vi "ReadAttribute_YCC.vi"() -> ()   [LabVIEW 2014]
uses:
  <vilib>/vision/driver/IMAQdx.llb/IMAQdx Attribute Type.ctl
  <vilib>/vision/driver/IMAQdx.llb/IMAQdx Attribute Visibility.ctl
  <vilib>/userDefined/High Color/IMAQdx.ctl
  <vilib>/vision/driver/IMAQdx.llb/IMAQdx Camera Control Mode.ctl
  <vilib>/vision/driver/NI_Vision_Acquisition_Software.lvlib
  <resource>/objmgr/imaqdx.rc
panel:
  out "Array 2":string[](array[string])=["AcquisitionAttributes::AdvancedGenicam::CommandTimeout", "AcquisitionAttributes::AdvancedGenicam::EventQueueDepth", "AcquisitionAttributes::AdvancedGenicam::EventsEnabled", "AcquisitionAttributes::AdvancedGenicam::EventsSupported", "AcquisitionAttributes::AdvancedGenicam::IgnoreCameraValidationErrors", "AcquisitionAttributes::AdvancedUSB3Vision::ActualMaximumPayloadTransferSize", "AcquisitionAttributes::AdvancedUSB3Vision::RequiredPayloadSizeAlignment", "AcquisitionAttributes::Bayer::Algorithm", "AcquisitionAttributes::Bayer::GainB", "AcquisitionAttributes::Bayer::GainG", "AcquisitionAttributes::Bayer::GainR", "AcquisitionAttributes::Bayer::Pattern", "AcquisitionAttributes::ChunkDataDecoding::ChunkDataDecodingEnabled", "AcquisitionAttributes::ChunkDataDecoding::MaximumChunkCopySize", "CameraAttributes::SequencerControl::SequencerMode", "CameraAttributes::SequencerControl::SequencerSetActive", "CameraAttributes::SequencerControl::SequencerConfigurationMode", "CameraAttributes::SequencerControl::SequencerSetStart", "CameraAttributes::SequencerControl::SequencerSetSelector", "CameraAttributes::SequencerControl::SequencerSetLoad", "CameraAttributes::SequencerControl::SequencerSetSave", "CameraAttributes::SequencerControl::SequencerPathSelector", "CameraAttributes::SequencerControl::SequencerSetNext", "CameraAttributes::SequencerControl::SequencerTriggerSource", "CameraAttributes::SequencerControl::SequencerTriggerActivation", "CameraAttributes::ImageFormatControl::SensorWidth", "CameraAttributes::ImageFormatControl::SensorHeight", "CameraAttributes::ImageFormatControl::WidthMax", "CameraAttributes::ImageFormatControl::HeightMax", "CameraAttributes::ImageFormatControl::Width", "CameraAttributes::ImageFormatControl::Height", "CameraAttributes::ImageFormatControl::OffsetX", "CameraAttributes::ImageFormatControl::OffsetY", "CameraAttributes::ImageFormatControl::CenterX", "CameraAttributes::ImageFormatControl::CenterY", "CameraAttributes::ImageFormatControl::BinningHorizontalMode", "CameraAttributes::ImageFormatControl::BinningHorizontal", "CameraAttributes::ImageFormatControl::BinningVerticalMode", "CameraAttributes::ImageFormatControl::BinningVertical", "CameraAttributes::ImageFormatControl::ReverseX", "CameraAttributes::ImageFormatControl::ReverseY", "CameraAttributes::ImageFormatControl::PixelFormat", "CameraAttributes::ImageFormatControl::PixelSize", "CameraAttributes::ImageFormatControl::PixelColorFilter", "CameraAttributes::ImageFormatControl::PixelDynamicRangeMin", "CameraAttributes::ImageFormatControl::PixelDynamicRangeMax", "CameraAttributes::ImageFormatControl::TestImageSelector", "CameraAttributes::ImageFormatControl::TestImageResetAndHold", "CameraAttributes::ImageFormatControl::ROIZoneSelector", "CameraAttributes::ImageFormatControl::ROIZoneMode", "CameraAttributes::ImageFormatControl::ROIZoneSize", "CameraAttributes::ImageFormatControl::ROIZoneOffset", "CameraAttributes::AnalogControl::GainAuto", "CameraAttributes::AnalogControl::GainSelector", "CameraAttributes::AnalogControl::Gain", "CameraAttributes::AnalogControl::BlackLevelSelector", "CameraAttributes::AnalogControl::BlackLevel", "CameraAttributes::AnalogControl::Gamma", "CameraAttributes::AnalogControl::DigitalShift", "CameraAttributes::ImageQualityControl::PGIControl::PgiMode", "CameraAttributes::ImageQualityControl::PGIControl::NoiseReduction", "CameraAttributes::ImageQualityControl::PGIControl::SharpnessEnhancement", "CameraAttributes::ImageQualityControl::ColorTransformationValue", "CameraAttributes::AcquisitionControl::AcquisitionMode", "CameraAttributes::AcquisitionControl::ShutterMode", "CameraAttributes::AcquisitionControl::ExposureAuto", "CameraAttributes::AcquisitionControl::ExposureMode", "CameraAttributes::AcquisitionControl::ExposureTime", "CameraAttributes::AcquisitionControl::ExposureOverlapTimeMode", "CameraAttributes::AcquisitionControl::ExposureOverlapTimeMax", "CameraAttributes::AcquisitionControl::AcquisitionBurstFrameCount", "CameraAttributes::AcquisitionControl::TriggerSelector", "CameraAttributes::AcquisitionControl::TriggerMode", "CameraAttributes::AcquisitionControl::TriggerSoftware", "CameraAttributes::AcquisitionControl::TriggerSource", "CameraAttributes::AcquisitionControl::TriggerActivation", "CameraAttributes::AcquisitionControl::TriggerDelay", "CameraAttributes::AcquisitionControl::AcquisitionFrameRateEnable", "CameraAttributes::AcquisitionControl::AcquisitionFrameRate", "CameraAttributes::AcquisitionControl::ResultingFrameRate", "CameraAttributes::AcquisitionControl::SensorReadoutTime", "CameraAttributes::AcquisitionControl::AcquisitionStatusSelector", "CameraAttributes::AcquisitionControl::AcquisitionStatus", "CameraAttributes::AutoFunctionControl::AutoTargetBrightness", "CameraAttributes::AutoFunctionControl::AutoFunctionProfile", "CameraAttributes::AutoFunctionControl::AutoGainLowerLimit", "CameraAttributes::AutoFunctionControl::AutoGainUpperLimit", "CameraAttributes::AutoFunctionControl::AutoExposureTimeLowerLimit", "CameraAttributes::AutoFunctionControl::AutoExposureTimeUpperLimit", "CameraAttributes::AutoFunctionControl::AutoFunctionROIControl::AutoFunctionROISelector", "CameraAttributes::AutoFunctionControl::AutoFunctionROIControl::AutoFunctionROIWidth", "CameraAttributes::AutoFunctionControl::AutoFunctionROIControl::AutoFunctionROIHeight", "CameraAttributes::AutoFunctionControl::AutoFunctionROIControl::AutoFunctionROIOffsetX", "CameraAttributes::AutoFunctionControl::AutoFunctionROIControl::AutoFunctionROIOffsetY", "CameraAttributes::AutoFunctionControl::AutoFunctionROIControl::AutoFunctionROIUseBrightness", "CameraAttributes::AutoFunctionControl::AutoFunctionROIControl::AutoFunctionROIUseWhiteBalance", "CameraAttributes::LUTControl::LUTSelector", "CameraAttributes::LUTControl::LUTEnable", "CameraAttributes::LUTControl::LUTIndex", "CameraAttributes::LUTControl::LUTValue", "CameraAttributes::DigitalIOControl::LineSelector", "CameraAttributes::DigitalIOControl::LineMode", "CameraAttributes::DigitalIOControl::LineFormat", "CameraAttributes::DigitalIOControl::LineLogic", "CameraAttributes::DigitalIOControl::LineSource", "CameraAttributes::DigitalIOControl::LineInverter", "CameraAttributes::DigitalIOControl::LineDebouncerTime", "CameraAttributes::DigitalIOControl::LineMinimumOutputPulseWidth", "CameraAttributes::DigitalIOControl::LineOverloadStatus", "CameraAttributes::DigitalIOControl::LineStatus", "CameraAttributes::DigitalIOControl::LineStatusAll", "CameraAttributes::DigitalIOControl::UserOutputSelector", "CameraAttributes::DigitalIOControl::UserOutputValue", "CameraAttributes::DigitalIOControl::UserOutputValueAll", "CameraAttributes::SoftwareSignalControl::SoftwareSignalSelector", "CameraAttributes::SoftwareSignalControl::SoftwareSignalPulse", "CameraAttributes::CounterAndTimerControl::TimerSelector", "CameraAttributes::CounterAndTimerControl::TimerDuration", "CameraAttributes::CounterAndTimerControl::TimerDelay", "CameraAttributes::CounterAndTimerControl::TimerTriggerSource", "CameraAttributes::CounterAndTimerControl::CounterSelector", "CameraAttributes::CounterAndTimerControl::CounterEventSource", "CameraAttributes::CounterAndTimerControl::CounterResetSource", "CameraAttributes::CounterAndTimerControl::CounterResetActivation", "CameraAttributes::CounterAndTimerControl::CounterReset", "CameraAttributes::CounterAndTimerControl::CounterDuration", "CameraAttributes::ChunkDataControl::ChunkModeActive", "CameraAttributes::ChunkDataControl::ChunkSelector", "CameraAttributes::ChunkDataControl::ChunkEnable", "CameraAttributes::ChunkDataControl::ChunkGainSelector", "CameraAttributes::ChunkDataControl::ChunkGain", "CameraAttributes::ChunkDataControl::ChunkExposureTime", "CameraAttributes::ChunkDataControl::ChunkTimestamp", "CameraAttributes::ChunkDataControl::ChunkLineStatusAll", "CameraAttributes::ChunkDataControl::ChunkCounterSelector", "CameraAttributes::ChunkDataControl::ChunkCounterValue", "CameraAttributes::ChunkDataControl::ChunkSequencerSetActive", "CameraAttributes::ChunkDataControl::ChunkPayloadCRC16", "CameraAttributes::ChunkDataControl::ChunkData::ChunkGainSelector", "CameraAttributes::ChunkDataControl::ChunkData::ChunkGain", "CameraAttributes::ChunkDataControl::ChunkData::ChunkExposureTime", "CameraAttributes::ChunkDataControl::ChunkData::ChunkTimestamp", "CameraAttributes::ChunkDataControl::ChunkData::ChunkLineStatusAll", "CameraAttributes::ChunkDataControl::ChunkData::ChunkCounterSelector", "CameraAttributes::ChunkDataControl::ChunkData::ChunkCounterValue", "CameraAttributes::ChunkDataControl::ChunkData::ChunkSequencerSetActive", "CameraAttributes::ChunkDataControl::ChunkData::ChunkPayloadCRC16", "CameraAttributes::EventControl::EventSelector", "CameraAttributes::EventControl::EventNotification", "CameraAttributes::EventControl::EventExposureEndData::EventExposureEnd", "CameraAttributes::EventControl::EventExposureEndData::EventExposureEndTimestamp", "CameraAttributes::EventControl::EventExposureEndData::EventExposureEndFrameID", "CameraAttributes::EventControl::EventFrameStartData::EventFrameStart", "CameraAttributes::EventControl::EventFrameStartData::EventFrameStartTimestamp", "CameraAttributes::EventControl::EventFrameStartData::EventFrameStartFrameID", "CameraAttributes::EventControl::EventFrameBurstStartData::EventFrameBurstStart", "CameraAttributes::EventControl::EventFrameBurstStartData::EventFrameBurstStartTimestamp", "CameraAttributes::EventControl::EventFrameBurstStartData::EventFrameBurstStartFrameID", "CameraAttributes::EventControl::EventFrameStartOvertriggerData::EventFrameStartOvertrigger", "CameraAttributes::EventControl::EventFrameStartOvertriggerData::EventFrameStartOvertriggerTimestamp", "CameraAttributes::EventControl::EventFrameStartOvertriggerData::EventFrameStartOvertriggerFrameID", "CameraAttributes::EventControl::EventFrameBurstStartOvertriggerData::EventFrameBurstStartOvertrigger", "CameraAttributes::EventControl::EventFrameBurstStartOvertriggerData::EventFrameBurstStartOvertriggerTimestamp", "CameraAttributes::EventControl::EventFrameBurstStartOvertriggerData::EventFrameBurstStartOvertriggerFrameID", "CameraAttributes::EventControl::EventCriticalTemperatureData::EventCriticalTemperature", "CameraAttributes::EventControl::EventCriticalTemperatureData::EventCriticalTemperatureTimestamp", "CameraAttributes::EventControl::EventOverTemperatureData::EventOverTemperature", "CameraAttributes::EventControl::EventOverTemperatureData::EventOverTemperatureTimestamp", "CameraAttributes::EventControl::EventFrameStartWaitData::EventFrameStartWait", "CameraAttributes::EventControl::EventFrameStartWaitData::EventFrameStartWaitTimestamp", "CameraAttributes::EventControl::EventFrameBurstStartWaitData::EventFrameBurstStartWait", "CameraAttributes::EventControl::EventFrameBurstStartWaitData::EventFrameBurstStartWaitTimestamp", "CameraAttributes::UserSetControl::UserSetSelector", "CameraAttributes::UserSetControl::UserSetLoad", "CameraAttributes::UserSetControl::UserSetSave", "CameraAttributes::UserSetControl::UserSetDefault", "CameraAttributes::TransportLayerControl::PayloadSize", "CameraAttributes::TransportLayerControl::BslUSBSpeedMode", "CameraAttributes::TransportLayerControl::SIPayloadTransferSize", "CameraAttributes::TransportLayerControl::SIPayloadTransferCount", "CameraAttributes::TransportLayerControl::SIPayloadFinalTransfer1Size", "CameraAttributes::TransportLayerControl::SIPayloadFinalTransfer2Size", "CameraAttributes::DeviceControl::DeviceVendorName", "CameraAttributes::DeviceControl::DeviceModelName", "CameraAttributes::DeviceControl::DeviceManufacturerInfo", "CameraAttributes::DeviceControl::DeviceVersion", "CameraAttributes::DeviceControl::DeviceFirmwareVersion", "CameraAttributes::DeviceControl::DeviceSerialNumber", "CameraAttributes::DeviceControl::DeviceUserID", "CameraAttributes::DeviceControl::DeviceScanType", "CameraAttributes::DeviceControl::TimestampLatch", "CameraAttributes::DeviceControl::TimestampLatchValue", "CameraAttributes::DeviceControl::DeviceLinkSelector", "CameraAttributes::DeviceControl::DeviceLinkSpeed", "CameraAttributes::DeviceControl::DeviceLinkThroughputLimitMode", "CameraAttributes::DeviceControl::DeviceLinkThroughputLimit", "CameraAttributes::DeviceControl::DeviceLinkCurrentThroughput", "CameraAttributes::DeviceControl::DeviceTemperatureSelector", "CameraAttributes::DeviceControl::DeviceTemperature", "CameraAttributes::DeviceControl::TemperatureState", "CameraAttributes::DeviceControl::DeviceSFNCVersionMajor", "CameraAttributes::DeviceControl::DeviceSFNCVersionMinor", "CameraAttributes::DeviceControl::DeviceSFNCVersionSubMinor", "CameraAttributes::UserDefinedValueControl::UserDefinedValueSelector", "CameraAttributes::UserDefinedValueControl::UserDefinedValue", "CameraAttributes::RemoveParameterLimitControl::RemoveParameterLimitSelector", "CameraAttributes::RemoveParameterLimitControl::RemoveParameterLimit", "CameraAttributes::ExpertFeatureAccess::ExpertFeatureAccessSelector", "CameraAttributes::ExpertFeatureAccess::ExpertFeatureAccessKey", "CameraAttributes::ExpertFeatureAccess::ExpertFeatureEnable", "CameraAttributes::FileAccessControl::FileSelector", "CameraAttributes::FileAccessControl::FileOperationSelector", "CameraAttributes::FileAccessControl::FileOpenMode", "CameraAttributes::FileAccessControl::FileAccessOffset", "CameraAttributes::FileAccessControl::FileAccessLength", "CameraAttributes::FileAccessControl::FileOperationStatus", "CameraAttributes::FileAccessControl::FileOperationResult", "CameraAttributes::FileAccessControl::FileSize", "CameraAttributes::FileAccessControl::FileOperationExecute", "AcquisitionAttributes::BitsPerPixel", "AcquisitionAttributes::ImageDecoderCopyMode", "AcquisitionAttributes::IncompleteBufferMode", "AcquisitionAttributes::OutputImageType", "AcquisitionAttributes::OverwriteMode", "AcquisitionAttributes::ReceiveTimestampMode", "AcquisitionAttributes::ShiftPixelBits", "AcquisitionAttributes::SwapPixelBytes", "AcquisitionAttributes::Timeout", "CameraInformation::BaseAddress", "CameraInformation::BusType", "CameraInformation::ModelName", "CameraInformation::PrimaryURLString", "CameraInformation::SecondaryURLString", "CameraInformation::SerialNumberHigh", "CameraInformation::SerialNumberLow", "CameraInformation::USBConnectionSpeed", "CameraInformation::VendorName", "StatusInformation::AcqInProgress", "StatusInformation::HandledEventCount", "StatusInformation::IncompleteBufferCount", "StatusInformation::LastBufferCount", "StatusInformation::LastBufferNumber", "StatusInformation::LostBufferCount", "StatusInformation::LostEventCount"]
  out "Writable name":string[](array[string])=["AcquisitionAttributes::AdvancedGenicam::EventQueueDepth", "AcquisitionAttributes::AdvancedGenicam::EventsEnabled", "AcquisitionAttributes::AdvancedGenicam::IgnoreCameraValidationErrors", "AcquisitionAttributes::Bayer::Algorithm", "AcquisitionAttributes::Bayer::GainB", "AcquisitionAttributes::Bayer::GainG", "AcquisitionAttributes::Bayer::GainR", "AcquisitionAttributes::Bayer::Pattern", "AcquisitionAttributes::ChunkDataDecoding::ChunkDataDecodingEnabled", "AcquisitionAttributes::ChunkDataDecoding::MaximumChunkCopySize", "AcquisitionAttributes::BitsPerPixel", "AcquisitionAttributes::ImageDecoderCopyMode", "AcquisitionAttributes::IncompleteBufferMode", "AcquisitionAttributes::OutputImageType", "AcquisitionAttributes::OverwriteMode", "AcquisitionAttributes::ReceiveTimestampMode", "AcquisitionAttributes::ShiftPixelBits", "AcquisitionAttributes::SwapPixelBytes", "AcquisitionAttributes::Timeout"]
  out "Attribute Information Array":T2(array[cluster])=[{"Attribute Type"=enum."U32", "Readable"=FALSE, "Writable"=FALSE, "Attribute Name"="AcquisitionAttributes::AdvancedGenicam::CommandTimeout"}, {"Attribute Type"=enum."U32", "Readable"=TRUE, "Writable"=TRUE, "Attribute Name"="AcquisitionAttributes::AdvancedGenicam::EventQueueDepth"}, {"Attribute Type"=enum."Bool", "Readable"=TRUE, "Writable"=TRUE, "Attribute Name"="AcquisitionAttributes::AdvancedGenicam::EventsEnabled"}, {"Attribute Type"=enum."Bool", "Readable"=TRUE, "Writable"=FALSE, "Attribute Name"="AcquisitionAttributes::AdvancedGenicam::EventsSupported"}, {"Attribute Type"=enum."Bool", "Readable"=TRUE, "Writable"=TRUE, "Attribute Name"="AcquisitionAttributes::AdvancedGenicam::IgnoreCameraValidationErrors"}, {"Attribute Type"=enum."U32", "Readable"=TRUE, "Writable"=FALSE, "Attribute Name"="AcquisitionAttributes::AdvancedUSB3Vision::ActualMaximumPayloadTransferSize"}, {"Attribute Type"=enum."U32", "Readable"=TRUE, "Writable"=FALSE, "Attribute Name"="AcquisitionAttributes::AdvancedUSB3Vision::RequiredPayloadSizeAlignment"}, {"Attribute Type"=enum."Enum", "Readable"=TRUE, "Writable"=TRUE, "Attribute Name"="AcquisitionAttributes::Bayer::Algorithm"}, {"Attribute Type"=enum."DBL", "Readable"=TRUE, "Writable"=TRUE, "Attribute Name"="AcquisitionAttributes::Bayer::GainB"}, {"Attribute Type"=enum."DBL", "Readable"=TRUE, "Writable"=TRUE, "Attribute Name"="AcquisitionAttributes::Bayer::GainG"}, {"Attribute Type"=enum."DBL", "Readable"=TRUE, "Writable"=TRUE, "Attribute Name"="AcquisitionAttributes::Bayer::GainR"}, {"Attribute Type"=enum."Enum", "Readable"=TRUE, "Writable"=TRUE, "Attribute Name"="AcquisitionAttributes::Bayer::Pattern"}, {"Attribute Type"=enum."Bool", "Readable"=TRUE, "Writable"=TRUE, "Attribute Name"="AcquisitionAttributes::ChunkDataDecoding::ChunkDataDecodingEnabled"}, {"Attribute Type"=enum."U32", "Readable"=TRUE, "Writable"=TRUE, "Attribute Name"="AcquisitionAttributes::ChunkDataDecoding::MaximumChunkCopySize"}, {"Attribute Type"=enum."Enum", "Readable"=TRUE, "Writable"=FALSE, "Attribute Name"="CameraAttributes::SequencerControl::SequencerMode"}, {"Attribute Type"=enum."I64", "Readable"=FALSE, "Writable"=FALSE, "Attribute Name"="CameraAttributes::SequencerControl::SequencerSetActive"}, {"Attribute Type"=enum."Enum", "Readable"=TRUE, "Writable"=FALSE, "Attribute Name"="CameraAttributes::SequencerControl::SequencerConfigurationMode"}, {"Attribute Type"=enum."I64", "Readable"=TRUE, "Writable"=FALSE, "Attribute Name"="CameraAttributes::SequencerControl::SequencerSetStart"}, {"Attribute Type"=enum."I64", "Readable"=TRUE, "Writable"=FALSE, "Attribute Name"="CameraAttributes::SequencerControl::SequencerSetSelector"}, {"Attribute Type"=enum."Command", "Readable"=FALSE, "Writable"=FALSE, "Attribute Name"="CameraAttributes::SequencerControl::SequencerSetLoad"}, {"Attribute Type"=enum."Command", "Readable"=FALSE, "Writable"=FALSE, "Attribute Name"="CameraAttributes::SequencerControl::SequencerSetSave"}, {"Attribute Type"=enum."I64", "Readable"=TRUE, "Writable"=FALSE, "Attribute Name"="CameraAttributes::SequencerControl::SequencerPathSelector"}, {"Attribute Type"=enum."I64", "Readable"=TRUE, "Writable"=FALSE, "Attribute Name"="CameraAttributes::SequencerControl::SequencerSetNext"}, {"Attribute Type"=enum."Enum", "Readable"=TRUE, "Writable"=FALSE, "Attribute Name"="CameraAttributes::SequencerControl::SequencerTriggerSource"}, {"Attribute Type"=enum."Enum", "Readable"=TRUE, "Writable"=FALSE, "Attribute Name"="CameraAttributes::SequencerControl::SequencerTriggerActivation"}, {"Attribute Type"=enum."I64", "Readable"=TRUE, "Writable"=FALSE, "Attribute Name"="CameraAttributes::ImageFormatControl::SensorWidth"}, {"Attribute Type"=enum."I64", "Readable"=TRUE, "Writable"=FALSE, "Attribute Name"="CameraAttributes::ImageFormatControl::SensorHeight"}, {"Attribute Type"=enum."I64", "Readable"=TRUE, "Writable"=FALSE, "Attribute Name"="CameraAttributes::ImageFormatControl::WidthMax"}, {"Attribute Type"=enum."I64", "Readable"=TRUE, "Writable"=FALSE, "Attribute Name"="CameraAttributes::ImageFormatControl::HeightMax"}, {"Attribute Type"=enum."I64", "Readable"=TRUE, "Writable"=FALSE, "Attribute Name"="CameraAttributes::ImageFormatControl::Width"}, {"Attribute Type"=enum."I64", "Readable"=TRUE, "Writable"=FALSE, "Attribute Name"="CameraAttributes::ImageFormatControl::Height"}, {"Attribute Type"=enum."I64", "Readable"=TRUE, "Writable"=FALSE, "Attribute Name"="CameraAttributes::ImageFormatControl::OffsetX"}, {"Attribute Type"=enum."I64", "Readable"=TRUE, "Writable"=FALSE, "Attribute Name"="CameraAttributes::ImageFormatControl::OffsetY"}, {"Attribute Type"=enum."Bool", "Readable"=TRUE, "Writable"=FALSE, "Attribute Name"="CameraAttributes::ImageFormatControl::CenterX"}, {"Attribute Type"=enum."Bool", "Readable"=TRUE, "Writable"=FALSE, "Attribute Name"="CameraAttributes::ImageFormatControl::CenterY"}, {"Attribute Type"=enum."Enum", "Readable"=TRUE, "Writable"=FALSE, "Attribute Name"="CameraAttributes::ImageFormatControl::BinningHorizontalMode"}, {"Attribute Type"=enum."I64", "Readable"=TRUE, "Writable"=FALSE, "Attribute Name"="CameraAttributes::ImageFormatControl::BinningHorizontal"}, {"Attribute Type"=enum."Enum", "Readable"=TRUE, "Writable"=FALSE, "Attribute Name"="CameraAttributes::ImageFormatControl::BinningVerticalMode"}, {"Attribute Type"=enum."I64", "Readable"=TRUE, "Writable"=FALSE, "Attribute Name"="CameraAttributes::ImageFormatControl::BinningVertical"}, {"Attribute Type"=enum."Bool", "Readable"=TRUE, "Writable"=FALSE, "Attribute Name"="CameraAttributes::ImageFormatControl::ReverseX"}, {"Attribute Type"=enum."Bool", "Readable"=TRUE, "Writable"=FALSE, "Attribute Name"="CameraAttributes::ImageFormatControl::ReverseY"}, {"Attribute Type"=enum."Enum", "Readable"=TRUE, "Writable"=FALSE, "Attribute Name"="CameraAttributes::ImageFormatControl::PixelFormat"}, {"Attribute Type"=enum."Enum", "Readable"=TRUE, "Writable"=FALSE, "Attribute Name"="CameraAttributes::ImageFormatControl::PixelSize"}, {"Attribute Type"=enum."Enum", "Readable"=TRUE, "Writable"=FALSE, "Attribute Name"="CameraAttributes::ImageFormatControl::PixelColorFilter"}, {"Attribute Type"=enum."I64", "Readable"=TRUE, "Writable"=FALSE, "Attribute Name"="CameraAttributes::ImageFormatControl::PixelDynamicRangeMin"}, {"Attribute Type"=enum."I64", "Readable"=TRUE, "Writable"=FALSE, "Attribute Name"="CameraAttributes::ImageFormatControl::PixelDynamicRangeMax"}, {"Attribute Type"=enum."Enum", "Readable"=TRUE, "Writable"=FALSE, "Attribute Name"="CameraAttributes::ImageFormatControl::TestImageSelector"}, {"Attribute Type"=enum."Bool", "Readable"=TRUE, "Writable"=FALSE, "Attribute Name"="CameraAttributes::ImageFormatControl::TestImageResetAndHold"}, {"Attribute Type"=enum."Enum", "Readable"=TRUE, "Writable"=FALSE, "Attribute Name"="CameraAttributes::ImageFormatControl::ROIZoneSelector"}, {"Attribute Type"=enum."Enum", "Readable"=TRUE, "Writable"=FALSE, "Attribute Name"="CameraAttributes::ImageFormatControl::ROIZoneMode"}, {"Attribute Type"=enum."I64", "Readable"=TRUE, "Writable"=FALSE, "Attribute Name"="CameraAttributes::ImageFormatControl::ROIZoneSize"}, {"Attribute Type"=enum."I64", "Readable"=TRUE, "Writable"=FALSE, "Attribute Name"="CameraAttributes::ImageFormatControl::ROIZoneOffset"}, {"Attribute Type"=enum."Enum", "Readable"=TRUE, "Writable"=FALSE, "Attribute Name"="CameraAttributes::AnalogControl::GainAuto"}, {"Attribute Type"=enum."Enum", "Readable"=TRUE, "Writable"=FALSE, "Attribute Name"="CameraAttributes::AnalogControl::GainSelector"}, {"Attribute Type"=enum."DBL", "Readable"=TRUE, "Writable"=FALSE, "Attribute Name"="CameraAttributes::AnalogControl::Gain"}, {"Attribute Type"=enum."Enum", "Readable"=TRUE, "Writable"=FALSE, "Attribute Name"="CameraAttributes::AnalogControl::BlackLevelSelector"}, {"Attribute Type"=enum."DBL", "Readable"=TRUE, "Writable"=FALSE, "Attribute Name"="CameraAttributes::AnalogControl::BlackLevel"}, {"Attribute Type"=enum."DBL", "Readable"=TRUE, "Writable"=FALSE, "Attribute Name"="CameraAttributes::AnalogControl::Gamma"}, {"Attribute Type"=enum."I64", "Readable"=TRUE, "Writable"=FALSE, "Attribute Name"="CameraAttributes::AnalogControl::DigitalShift"}, {"Attribute Type"=enum."Enum", "Readable"=TRUE, "Writable"=FALSE, "Attribute Name"="CameraAttributes::ImageQualityControl::PGIControl::PgiMode"}, {"Attribute Type"=enum."DBL", "Readable"=FALSE, "Writable"=FALSE, "Attribute Name"="CameraAttributes::ImageQualityControl::PGIControl::NoiseReduction"}, {"Attribute Type"=enum."DBL", "Readable"=FALSE, "Writable"=FALSE, "Attribute Name"="CameraAttributes::ImageQualityControl::PGIControl::SharpnessEnhancement"}, {"Attribute Type"=enum."DBL", "Readable"=FALSE, "Writable"=FALSE, "Attribute Name"="CameraAttributes::ImageQualityControl::ColorTransformationValue"}, {"Attribute Type"=enum."Enum", "Readable"=TRUE, "Writable"=FALSE, "Attribute Name"="CameraAttributes::AcquisitionControl::AcquisitionMode"}, {"Attribute Type"=enum."Enum", "Readable"=TRUE, "Writable"=FALSE, "Attribute Name"="CameraAttributes::AcquisitionControl::ShutterMode"}, {"Attribute Type"=enum."Enum", "Readable"=TRUE, "Writable"=FALSE, "Attribute Name"="CameraAttributes::AcquisitionControl::ExposureAuto"}, {"Attribute Type"=enum."Enum", "Readable"=TRUE, "Writable"=FALSE, "Attribute Name"="CameraAttributes::AcquisitionControl::ExposureMode"}, {"Attribute Type"=enum."DBL", "Readable"=TRUE, "Writable"=FALSE, "Attribute Name"="CameraAttributes::AcquisitionControl::ExposureTime"}, {"Attribute Type"=enum."Enum", "Readable"=FALSE, "Writable"=FALSE, "Attribute Name"="CameraAttributes::AcquisitionControl::ExposureOverlapTimeMode"}, {"Attribute Type"=enum."DBL", "Readable"=FALSE, "Writable"=FALSE, "Attribute Name"="CameraAttributes::AcquisitionControl::ExposureOverlapTimeMax"}, {"Attribute Type"=enum."I64", "Readable"=TRUE, "Writable"=FALSE, "Attribute Name"="CameraAttributes::AcquisitionControl::AcquisitionBurstFrameCount"}, {"Attribute Type"=enum."Enum", "Readable"=TRUE, "Writable"=FALSE, "Attribute Name"="CameraAttributes::AcquisitionControl::TriggerSelector"}, {"Attribute Type"=enum."Enum", "Readable"=TRUE, "Writable"=FALSE, "Attribute Name"="CameraAttributes::AcquisitionControl::TriggerMode"}, {"Attribute Type"=enum."Command", "Readable"=FALSE, "Writable"=FALSE, "Attribute Name"="CameraAttributes::AcquisitionControl::TriggerSoftware"}, {"Attribute Type"=enum."Enum", "Readable"=TRUE, "Writable"=FALSE, "Attribute Name"="CameraAttributes::AcquisitionControl::TriggerSource"}, {"Attribute Type"=enum."Enum", "Readable"=TRUE, "Writable"=FALSE, "Attribute Name"="CameraAttributes::AcquisitionControl::TriggerActivation"}, {"Attribute Type"=enum."DBL", "Readable"=TRUE, "Writable"=FALSE, "Attribute Name"="CameraAttributes::AcquisitionControl::TriggerDelay"}, {"Attribute Type"=enum."Bool", "Readable"=TRUE, "Writable"=FALSE, "Attribute Name"="CameraAttributes::AcquisitionControl::AcquisitionFrameRateEnable"}, {"Attribute Type"=enum."DBL", "Readable"=TRUE, "Writable"=FALSE, "Attribute Name"="CameraAttributes::AcquisitionControl::AcquisitionFrameRate"}, {"Attribute Type"=enum."DBL", "Readable"=TRUE, "Writable"=FALSE, "Attribute Name"="CameraAttributes::AcquisitionControl::ResultingFrameRate"}, {"Attribute Type"=enum."DBL", "Readable"=TRUE, "Writable"=FALSE, "Attribute Name"="CameraAttributes::AcquisitionControl::SensorReadoutTime"}, {"Attribute Type"=enum."Enum", "Readable"=TRUE, "Writable"=FALSE, "Attribute Name"="CameraAttributes::AcquisitionControl::AcquisitionStatusSelector"}, {"Attribute Type"=enum."Bool", "Readable"=TRUE, "Writable"=FALSE, "Attribute Name"="CameraAttributes::AcquisitionControl::AcquisitionStatus"}, {"Attribute Type"=enum."DBL", "Readable"=TRUE, "Writable"=FALSE, "Attribute Name"="CameraAttributes::AutoFunctionControl::AutoTargetBrightness"}, {"Attribute Type"=enum."Enum", "Readable"=TRUE, "Writable"=FALSE, "Attribute Name"="CameraAttributes::AutoFunctionControl::AutoFunctionProfile"}, {"Attribute Type"=enum."DBL", "Readable"=TRUE, "Writable"=FALSE, "Attribute Name"="CameraAttributes::AutoFunctionControl::AutoGainLowerLimit"}, {"Attribute Type"=enum."DBL", "Readable"=TRUE, "Writable"=FALSE, "Attribute Name"="CameraAttributes::AutoFunctionControl::AutoGainUpperLimit"}, {"Attribute Type"=enum."DBL", "Readable"=TRUE, "Writable"=FALSE, "Attribute Name"="CameraAttributes::AutoFunctionControl::AutoExposureTimeLowerLimit"}, {"Attribute Type"=enum."DBL", "Readable"=TRUE, "Writable"=FALSE, "Attribute Name"="CameraAttributes::AutoFunctionControl::AutoExposureTimeUpperLimit"}, {"Attribute Type"=enum."Enum", "Readable"=TRUE, "Writable"=FALSE, "Attribute Name"="CameraAttributes::AutoFunctionControl::AutoFunctionROIControl::AutoFunctionROISelector"}, {"Attribute Type"=enum."I64", "Readable"=TRUE, "Writable"=FALSE, "Attribute Name"="CameraAttributes::AutoFunctionControl::AutoFunctionROIControl::AutoFunctionROIWidth"}, {"Attribute Type"=enum."I64", "Readable"=TRUE, "Writable"=FALSE, "Attribute Name"="CameraAttributes::AutoFunctionControl::AutoFunctionROIControl::AutoFunctionROIHeight"}, {"Attribute Type"=enum."I64", "Readable"=TRUE, "Writable"=FALSE, "Attribute Name"="CameraAttributes::AutoFunctionControl::AutoFunctionROIControl::AutoFunctionROIOffsetX"}, {"Attribute Type"=enum."I64", "Readable"=TRUE, "Writable"=FALSE, "Attribute Name"="CameraAttributes::AutoFunctionControl::AutoFunctionROIControl::AutoFunctionROIOffsetY"}, {"Attribute Type"=enum."Bool", "Readable"=TRUE, "Writable"=FALSE, "Attribute Name"="CameraAttributes::AutoFunctionControl::AutoFunctionROIControl::AutoFunctionROIUseBrightness"}, {"Attribute Type"=enum."Bool", "Readable"=TRUE, "Writable"=FALSE, "Attribute Name"="CameraAttributes::AutoFunctionControl::AutoFunctionROIControl::AutoFunctionROIUseWhiteBalance"}, {"Attribute Type"=enum."Enum", "Readable"=TRUE, "Writable"=FALSE, "Attribute Name"="CameraAttributes::LUTControl::LUTSelector"}, {"Attribute Type"=enum."Bool", "Readable"=TRUE, "Writable"=FALSE, "Attribute Name"="CameraAttributes::LUTControl::LUTEnable"}, {"Attribute Type"=enum."I64", "Readable"=TRUE, "Writable"=FALSE, "Attribute Name"="CameraAttributes::LUTControl::LUTIndex"}, {"Attribute Type"=enum."I64", "Readable"=TRUE, "Writable"=FALSE, "Attribute Name"="CameraAttributes::LUTControl::LUTValue"}, {"Attribute Type"=enum."Enum", "Readable"=TRUE, "Writable"=FALSE, "Attribute Name"="CameraAttributes::DigitalIOControl::LineSelector"}, {"Attribute Type"=enum."Enum", "Readable"=TRUE, "Writable"=FALSE, "Attribute Name"="CameraAttributes::DigitalIOControl::LineMode"}, {"Attribute Type"=enum."Enum", "Readable"=TRUE, "Writable"=FALSE, "Attribute Name"="CameraAttributes::DigitalIOControl::LineFormat"}, {"Attribute Type"=enum."Enum", "Readable"=TRUE, "Writable"=FALSE, "Attribute Name"="CameraAttributes::DigitalIOControl::LineLogic"}, {"Attribute Type"=enum."Enum", "Readable"=FALSE, "Writable"=FALSE, "Attribute Name"="CameraAttributes::DigitalIOControl::LineSource"}, {"Attribute Type"=enum."Bool", "Readable"=TRUE, "Writable"=FALSE, "Attribute Name"="CameraAttributes::DigitalIOControl::LineInverter"}, {"Attribute Type"=enum."DBL", "Readable"=TRUE, "Writable"=FALSE, "Attribute Name"="CameraAttributes::DigitalIOControl::LineDebouncerTime"}, {"Attribute Type"=enum."DBL", "Readable"=FALSE, "Writable"=FALSE, "Attribute Name"="CameraAttributes::DigitalIOControl::LineMinimumOutputPulseWidth"}, {"Attribute Type"=enum."Bool", "Readable"=FALSE, "Writable"=FALSE, "Attribute Name"="CameraAttributes::DigitalIOControl::LineOverloadStatus"}, {"Attribute Type"=enum."Bool", "Readable"=TRUE, "Writable"=FALSE, "Attribute Name"="CameraAttributes::DigitalIOControl::LineStatus"}, {"Attribute Type"=enum."I64", "Readable"=TRUE, "Writable"=FALSE, "Attribute Name"="CameraAttributes::DigitalIOControl::LineStatusAll"}, {"Attribute Type"=enum."Enum", "Readable"=TRUE, "Writable"=FALSE, "Attribute Name"="CameraAttributes::DigitalIOControl::UserOutputSelector"}, {"Attribute Type"=enum."Bool", "Readable"=TRUE, "Writable"=FALSE, "Attribute Name"="CameraAttributes::DigitalIOControl::UserOutputValue"}, {"Attribute Type"=enum."I64", "Readable"=TRUE, "Writable"=FALSE, "Attribute Name"="CameraAttributes::DigitalIOControl::UserOutputValueAll"}, {"Attribute Type"=enum."Enum", "Readable"=TRUE, "Writable"=FALSE, "Attribute Name"="CameraAttributes::SoftwareSignalControl::SoftwareSignalSelector"}, {"Attribute Type"=enum."Command", "Readable"=FALSE, "Writable"=FALSE, "Attribute Name"="CameraAttributes::SoftwareSignalControl::SoftwareSignalPulse"}, {"Attribute Type"=enum."Enum", "Readable"=TRUE, "Writable"=FALSE, "Attribute Name"="CameraAttributes::CounterAndTimerControl::TimerSelector"}, {"Attribute Type"=enum."DBL", "Readable"=TRUE, "Writable"=FALSE, "Attribute Name"="CameraAttributes::CounterAndTimerControl::TimerDuration"}, {"Attribute Type"=enum."DBL", "Readable"=TRUE, "Writable"=FALSE, "Attribute Name"="CameraAttributes::CounterAndTimerControl::TimerDelay"}, {"Attribute Type"=enum."Enum", "Readable"=TRUE, "Writable"=FALSE, "Attribute Name"="CameraAttributes::CounterAndTimerControl::TimerTriggerSource"}, {"Attribute Type"=enum."Enum", "Readable"=TRUE, "Writable"=FALSE, "Attribute Name"="CameraAttributes::CounterAndTimerControl::CounterSelector"}, {"Attribute Type"=enum."Enum", "Readable"=TRUE, "Writable"=FALSE, "Attribute Name"="CameraAttributes::CounterAndTimerControl::CounterEventSource"}, {"Attribute Type"=enum."Enum", "Readable"=TRUE, "Writable"=FALSE, "Attribute Name"="CameraAttributes::CounterAndTimerControl::CounterResetSource"}, {"Attribute Type"=enum."Enum", "Readable"=TRUE, "Writable"=FALSE, "Attribute Name"="CameraAttributes::CounterAndTimerControl::CounterResetActivation"}, {"Attribute Type"=enum."Command", "Readable"=FALSE, "Writable"=FALSE, "Attribute Name"="CameraAttributes::CounterAndTimerControl::CounterReset"}, {"Attribute Type"=enum."I64", "Readable"=FALSE, "Writable"=FALSE, "Attribute Name"="CameraAttributes::CounterAndTimerControl::CounterDuration"}, {"Attribute Type"=enum."Bool", "Readable"=TRUE, "Writable"=FALSE, "Attribute Name"="CameraAttributes::ChunkDataControl::ChunkModeActive"}, {"Attribute Type"=enum."Enum", "Readable"=TRUE, "Writable"=FALSE, "Attribute Name"="CameraAttributes::ChunkDataControl::ChunkSelector"}, {"Attribute Type"=enum."Bool", "Readable"=TRUE, "Writable"=FALSE, "Attribute Name"="CameraAttributes::ChunkDataControl::ChunkEnable"}, {"Attribute Type"=enum."Enum", "Readable"=FALSE, "Writable"=FALSE, "Attribute Name"="CameraAttributes::ChunkDataControl::ChunkGainSelector"}, {"Attribute Type"=enum."DBL", "Readable"=FALSE, "Writable"=FALSE, "Attribute Name"="CameraAttributes::ChunkDataControl::ChunkGain"}, {"Attribute Type"=enum."DBL", "Readable"=FALSE, "Writable"=FALSE, "Attribute Name"="CameraAttributes::ChunkDataControl::ChunkExposureTime"}, {"Attribute Type"=enum."I64", "Readable"=FALSE, "Writable"=FALSE, "Attribute Name"="CameraAttributes::ChunkDataControl::ChunkTimestamp"}, {"Attribute Type"=enum."I64", "Readable"=FALSE, "Writable"=FALSE, "Attribute Name"="CameraAttributes::ChunkDataControl::ChunkLineStatusAll"}, {"Attribute Type"=enum."Enum", "Readable"=FALSE, "Writable"=FALSE, "Attribute Name"="CameraAttributes::ChunkDataControl::ChunkCounterSelector"}, {"Attribute Type"=enum."I64", "Readable"=FALSE, "Writable"=FALSE, "Attribute Name"="CameraAttributes::ChunkDataControl::ChunkCounterValue"}, {"Attribute Type"=enum."I64", "Readable"=FALSE, "Writable"=FALSE, "Attribute Name"="CameraAttributes::ChunkDataControl::ChunkSequencerSetActive"}, {"Attribute Type"=enum."I64", "Readable"=FALSE, "Writable"=FALSE, "Attribute Name"="CameraAttributes::ChunkDataControl::ChunkPayloadCRC16"}, {"Attribute Type"=enum."Enum", "Readable"=FALSE, "Writable"=FALSE, "Attribute Name"="CameraAttributes::ChunkDataControl::ChunkData::ChunkGainSelector"}, {"Attribute Type"=enum."DBL", "Readable"=FALSE, "Writable"=FALSE, "Attribute Name"="CameraAttributes::ChunkDataControl::ChunkData::ChunkGain"}, {"Attribute Type"=enum."DBL", "Readable"=FALSE, "Writable"=FALSE, "Attribute Name"="CameraAttributes::ChunkDataControl::ChunkData::ChunkExposureTime"}, {"Attribute Type"=enum."I64", "Readable"=FALSE, "Writable"=FALSE, "Attribute Name"="CameraAttributes::ChunkDataControl::ChunkData::ChunkTimestamp"}, {"Attribute Type"=enum."I64", "Readable"=FALSE, "Writable"=FALSE, "Attribute Name"="CameraAttributes::ChunkDataControl::ChunkData::ChunkLineStatusAll"}, {"Attribute Type"=enum."Enum", "Readable"=FALSE, "Writable"=FALSE, "Attribute Name"="CameraAttributes::ChunkDataControl::ChunkData::ChunkCounterSelector"}, {"Attribute Type"=enum."I64", "Readable"=FALSE, "Writable"=FALSE, "Attribute Name"="CameraAttributes::ChunkDataControl::ChunkData::ChunkCounterValue"}, {"Attribute Type"=enum."I64", "Readable"=FALSE, "Writable"=FALSE, "Attribute Name"="CameraAttributes::ChunkDataControl::ChunkData::ChunkSequencerSetActive"}, {"Attribute Type"=enum."I64", "Readable"=FALSE, "Writable"=FALSE, "Attribute Name"="CameraAttributes::ChunkDataControl::ChunkData::ChunkPayloadCRC16"}, {"Attribute Type"=enum."Enum", "Readable"=TRUE, "Writable"=FALSE, "Attribute Name"="CameraAttributes::EventControl::EventSelector"}, {"Attribute Type"=enum."Enum", "Readable"=TRUE, "Writable"=FALSE, "Attribute Name"="CameraAttributes::EventControl::EventNotification"}, {"Attribute Type"=enum."I64", "Readable"=FALSE, "Writable"=FALSE, "Attribute Name"="CameraAttributes::EventControl::EventExposureEndData::EventExposureEnd"}, {"Attribute Type"=enum."I64", "Readable"=FALSE, "Writable"=FALSE, "Attribute Name"="CameraAttributes::EventControl::EventExposureEndData::EventExposureEndTimestamp"}, {"Attribute Type"=enum."I64", "Readable"=FALSE, "Writable"=FALSE, "Attribute Name"="CameraAttributes::EventControl::EventExposureEndData::EventExposureEndFrameID"}, {"Attribute Type"=enum."I64", "Readable"=FALSE, "Writable"=FALSE, "Attribute Name"="CameraAttributes::EventControl::EventFrameStartData::EventFrameStart"}, {"Attribute Type"=enum."I64", "Readable"=FALSE, "Writable"=FALSE, "Attribute Name"="CameraAttributes::EventControl::EventFrameStartData::EventFrameStartTimestamp"}, {"Attribute Type"=enum."I64", "Readable"=FALSE, "Writable"=FALSE, "Attribute Name"="CameraAttributes::EventControl::EventFrameStartData::EventFrameStartFrameID"}, {"Attribute Type"=enum."I64", "Readable"=FALSE, "Writable"=FALSE, "Attribute Name"="CameraAttributes::EventControl::EventFrameBurstStartData::EventFrameBurstStart"}, {"Attribute Type"=enum."I64", "Readable"=FALSE, "Writable"=FALSE, "Attribute Name"="CameraAttributes::EventControl::EventFrameBurstStartData::EventFrameBurstStartTimestamp"}, {"Attribute Type"=enum."I64", "Readable"=FALSE, "Writable"=FALSE, "Attribute Name"="CameraAttributes::EventControl::EventFrameBurstStartData::EventFrameBurstStartFrameID"}, {"Attribute Type"=enum."I64", "Readable"=FALSE, "Writable"=FALSE, "Attribute Name"="CameraAttributes::EventControl::EventFrameStartOvertriggerData::EventFrameStartOvertrigger"}, {"Attribute Type"=enum."I64", "Readable"=FALSE, "Writable"=FALSE, "Attribute Name"="CameraAttributes::EventControl::EventFrameStartOvertriggerData::EventFrameStartOvertriggerTimestamp"}, {"Attribute Type"=enum."I64", "Readable"=FALSE, "Writable"=FALSE, "Attribute Name"="CameraAttributes::EventControl::EventFrameStartOvertriggerData::EventFrameStartOvertriggerFrameID"}, {"Attribute Type"=enum."I64", "Readable"=FALSE, "Writable"=FALSE, "Attribute Name"="CameraAttributes::EventControl::EventFrameBurstStartOvertriggerData::EventFrameBurstStartOvertrigger"}, {"Attribute Type"=enum."I64", "Readable"=FALSE, "Writable"=FALSE, "Attribute Name"="CameraAttributes::EventControl::EventFrameBurstStartOvertriggerData::EventFrameBurstStartOvertriggerTimestamp"}, {"Attribute Type"=enum."I64", "Readable"=FALSE, "Writable"=FALSE, "Attribute Name"="CameraAttributes::EventControl::EventFrameBurstStartOvertriggerData::EventFrameBurstStartOvertriggerFrameID"}, {"Attribute Type"=enum."I64", "Readable"=FALSE, "Writable"=FALSE, "Attribute Name"="CameraAttributes::EventControl::EventCriticalTemperatureData::EventCriticalTemperature"}, {"Attribute Type"=enum."I64", "Readable"=FALSE, "Writable"=FALSE, "Attribute Name"="CameraAttributes::EventControl::EventCriticalTemperatureData::EventCriticalTemperatureTimestamp"}, {"Attribute Type"=enum."I64", "Readable"=FALSE, "Writable"=FALSE, "Attribute Name"="CameraAttributes::EventControl::EventOverTemperatureData::EventOverTemperature"}, {"Attribute Type"=enum."I64", "Readable"=FALSE, "Writable"=FALSE, "Attribute Name"="CameraAttributes::EventControl::EventOverTemperatureData::EventOverTemperatureTimestamp"}, {"Attribute Type"=enum."I64", "Readable"=FALSE, "Writable"=FALSE, "Attribute Name"="CameraAttributes::EventControl::EventFrameStartWaitData::EventFrameStartWait"}, {"Attribute Type"=enum."I64", "Readable"=FALSE, "Writable"=FALSE, "Attribute Name"="CameraAttributes::EventControl::EventFrameStartWaitData::EventFrameStartWaitTimestamp"}, {"Attribute Type"=enum."I64", "Readable"=FALSE, "Writable"=FALSE, "Attribute Name"="CameraAttributes::EventControl::EventFrameBurstStartWaitData::EventFrameBurstStartWait"}, {"Attribute Type"=enum."I64", "Readable"=FALSE, "Writable"=FALSE, "Attribute Name"="CameraAttributes::EventControl::EventFrameBurstStartWaitData::EventFrameBurstStartWaitTimestamp"}, {"Attribute Type"=enum."Enum", "Readable"=TRUE, "Writable"=FALSE, "Attribute Name"="CameraAttributes::UserSetControl::UserSetSelector"}, {"Attribute Type"=enum."Command", "Readable"=FALSE, "Writable"=FALSE, "Attribute Name"="CameraAttributes::UserSetControl::UserSetLoad"}, {"Attribute Type"=enum."Command", "Readable"=FALSE, "Writable"=FALSE, "Attribute Name"="CameraAttributes::UserSetControl::UserSetSave"}, {"Attribute Type"=enum."Enum", "Readable"=TRUE, "Writable"=FALSE, "Attribute Name"="CameraAttributes::UserSetControl::UserSetDefault"}, {"Attribute Type"=enum."I64", "Readable"=TRUE, "Writable"=FALSE, "Attribute Name"="CameraAttributes::TransportLayerControl::PayloadSize"}, {"Attribute Type"=enum."Enum", "Readable"=TRUE, "Writable"=FALSE, "Attribute Name"="CameraAttributes::TransportLayerControl::BslUSBSpeedMode"}, {"Attribute Type"=enum."I64", "Readable"=TRUE, "Writable"=FALSE, "Attribute Name"="CameraAttributes::TransportLayerControl::SIPayloadTransferSize"}, {"Attribute Type"=enum."I64", "Readable"=TRUE, "Writable"=FALSE, "Attribute Name"="CameraAttributes::TransportLayerControl::SIPayloadTransferCount"}, {"Attribute Type"=enum."I64", "Readable"=TRUE, "Writable"=FALSE, "Attribute Name"="CameraAttributes::TransportLayerControl::SIPayloadFinalTransfer1Size"}, {"Attribute Type"=enum."I64", "Readable"=TRUE, "Writable"=FALSE, "Attribute Name"="CameraAttributes::TransportLayerControl::SIPayloadFinalTransfer2Size"}, {"Attribute Type"=enum."String", "Readable"=TRUE, "Writable"=FALSE, "Attribute Name"="CameraAttributes::DeviceControl::DeviceVendorName"}, {"Attribute Type"=enum."String", "Readable"=TRUE, "Writable"=FALSE, "Attribute Name"="CameraAttributes::DeviceControl::DeviceModelName"}, {"Attribute Type"=enum."String", "Readable"=TRUE, "Writable"=FALSE, "Attribute Name"="CameraAttributes::DeviceControl::DeviceManufacturerInfo"}, {"Attribute Type"=enum."String", "Readable"=TRUE, "Writable"=FALSE, "Attribute Name"="CameraAttributes::DeviceControl::DeviceVersion"}, {"Attribute Type"=enum."String", "Readable"=TRUE, "Writable"=FALSE, "Attribute Name"="CameraAttributes::DeviceControl::DeviceFirmwareVersion"}, {"Attribute Type"=enum."String", "Readable"=TRUE, "Writable"=FALSE, "Attribute Name"="CameraAttributes::DeviceControl::DeviceSerialNumber"}, {"Attribute Type"=enum."String", "Readable"=TRUE, "Writable"=FALSE, "Attribute Name"="CameraAttributes::DeviceControl::DeviceUserID"}, {"Attribute Type"=enum."Enum", "Readable"=TRUE, "Writable"=FALSE, "Attribute Name"="CameraAttributes::DeviceControl::DeviceScanType"}, {"Attribute Type"=enum."Command", "Readable"=FALSE, "Writable"=FALSE, "Attribute Name"="CameraAttributes::DeviceControl::TimestampLatch"}, {"Attribute Type"=enum."I64", "Readable"=TRUE, "Writable"=FALSE, "Attribute Name"="CameraAttributes::DeviceControl::TimestampLatchValue"}, {"Attribute Type"=enum."I64", "Readable"=TRUE, "Writable"=FALSE, "Attribute Name"="CameraAttributes::DeviceControl::DeviceLinkSelector"}, {"Attribute Type"=enum."I64", "Readable"=TRUE, "Writable"=FALSE, "Attribute Name"="CameraAttributes::DeviceControl::DeviceLinkSpeed"}, {"Attribute Type"=enum."Enum", "Readable"=TRUE, "Writable"=FALSE, "Attribute Name"="CameraAttributes::DeviceControl::DeviceLinkThroughputLimitMode"}, {"Attribute Type"=enum."I64", "Readable"=TRUE, "Writable"=FALSE, "Attribute Name"="CameraAttributes::DeviceControl::DeviceLinkThroughputLimit"}, {"Attribute Type"=enum."I64", "Readable"=TRUE, "Writable"=FALSE, "Attribute Name"="CameraAttributes::DeviceControl::DeviceLinkCurrentThroughput"}, {"Attribute Type"=enum."Enum", "Readable"=TRUE, "Writable"=FALSE, "Attribute Name"="CameraAttributes::DeviceControl::DeviceTemperatureSelector"}, {"Attribute Type"=enum."DBL", "Readable"=TRUE, "Writable"=FALSE, "Attribute Name"="CameraAttributes::DeviceControl::DeviceTemperature"}, {"Attribute Type"=enum."Enum", "Readable"=TRUE, "Writable"=FALSE, "Attribute Name"="CameraAttributes::DeviceControl::TemperatureState"}, {"Attribute Type"=enum."I64", "Readable"=TRUE, "Writable"=FALSE, "Attribute Name"="CameraAttributes::DeviceControl::DeviceSFNCVersionMajor"}, {"Attribute Type"=enum."I64", "Readable"=TRUE, "Writable"=FALSE, "Attribute Name"="CameraAttributes::DeviceControl::DeviceSFNCVersionMinor"}, {"Attribute Type"=enum."I64", "Readable"=TRUE, "Writable"=FALSE, "Attribute Name"="CameraAttributes::DeviceControl::DeviceSFNCVersionSubMinor"}, {"Attribute Type"=enum."Enum", "Readable"=TRUE, "Writable"=FALSE, "Attribute Name"="CameraAttributes::UserDefinedValueControl::UserDefinedValueSelector"}, {"Attribute Type"=enum."I64", "Readable"=TRUE, "Writable"=FALSE, "Attribute Name"="CameraAttributes::UserDefinedValueControl::UserDefinedValue"}, {"Attribute Type"=enum."Enum", "Readable"=TRUE, "Writable"=FALSE, "Attribute Name"="CameraAttributes::RemoveParameterLimitControl::RemoveParameterLimitSelector"}, {"Attribute Type"=enum."Bool", "Readable"=TRUE, "Writable"=FALSE, "Attribute Name"="CameraAttributes::RemoveParameterLimitControl::RemoveParameterLimit"}, {"Attribute Type"=enum."Enum", "Readable"=TRUE, "Writable"=FALSE, "Attribute Name"="CameraAttributes::ExpertFeatureAccess::ExpertFeatureAccessSelector"}, {"Attribute Type"=enum."I64", "Readable"=TRUE, "Writable"=FALSE, "Attribute Name"="CameraAttributes::ExpertFeatureAccess::ExpertFeatureAccessKey"}, {"Attribute Type"=enum."Bool", "Readable"=FALSE, "Writable"=FALSE, "Attribute Name"="CameraAttributes::ExpertFeatureAccess::ExpertFeatureEnable"}, {"Attribute Type"=enum."Enum", "Readable"=TRUE, "Writable"=FALSE, "Attribute Name"="CameraAttributes::FileAccessControl::FileSelector"}, {"Attribute Type"=enum."Enum", "Readable"=TRUE, "Writable"=FALSE, "Attribute Name"="CameraAttributes::FileAccessControl::FileOperationSelector"}, {"Attribute Type"=enum."Enum", "Readable"=TRUE, "Writable"=FALSE, "Attribute Name"="CameraAttributes::FileAccessControl::FileOpenMode"}, {"Attribute Type"=enum."I64", "Readable"=TRUE, "Writable"=FALSE, "Attribute Name"="CameraAttributes::FileAccessControl::FileAccessOffset"}, {"Attribute Type"=enum."I64", "Readable"=TRUE, "Writable"=FALSE, "Attribute Name"="CameraAttributes::FileAccessControl::FileAccessLength"}, {"Attribute Type"=enum."Enum", "Readable"=TRUE, "Writable"=FALSE, "Attribute Name"="CameraAttributes::FileAccessControl::FileOperationStatus"}, {"Attribute Type"=enum."I64", "Readable"=TRUE, "Writable"=FALSE, "Attribute Name"="CameraAttributes::FileAccessControl::FileOperationResult"}, {"Attribute Type"=enum."I64", "Readable"=TRUE, "Writable"=FALSE, "Attribute Name"="CameraAttributes::FileAccessControl::FileSize"}, {"Attribute Type"=enum."Command", "Readable"=FALSE, "Writable"=FALSE, "Attribute Name"="CameraAttributes::FileAccessControl::FileOperationExecute"}, {"Attribute Type"=enum."Enum", "Readable"=TRUE, "Writable"=TRUE, "Attribute Name"="AcquisitionAttributes::BitsPerPixel"}, {"Attribute Type"=enum."Enum", "Readable"=TRUE, "Writable"=TRUE, "Attribute Name"="AcquisitionAttributes::ImageDecoderCopyMode"}, {"Attribute Type"=enum."Enum", "Readable"=TRUE, "Writable"=TRUE, "Attribute Name"="AcquisitionAttributes::IncompleteBufferMode"}, {"Attribute Type"=enum."Enum", "Readable"=TRUE, "Writable"=TRUE, "Attribute Name"="AcquisitionAttributes::OutputImageType"}, {"Attribute Type"=enum."Enum", "Readable"=TRUE, "Writable"=TRUE, "Attribute Name"="AcquisitionAttributes::OverwriteMode"}, {"Attribute Type"=enum."Enum", "Readable"=TRUE, "Writable"=TRUE, "Attribute Name"="AcquisitionAttributes::ReceiveTimestampMode"}, {"Attribute Type"=enum."Bool", "Readable"=TRUE, "Writable"=TRUE, "Attribute Name"="AcquisitionAttributes::ShiftPixelBits"}, {"Attribute Type"=enum."Bool", "Readable"=TRUE, "Writable"=TRUE, "Attribute Name"="AcquisitionAttributes::SwapPixelBytes"}, {"Attribute Type"=enum."U32", "Readable"=TRUE, "Writable"=TRUE, "Attribute Name"="AcquisitionAttributes::Timeout"}, {"Attribute Type"=enum."U32", "Readable"=TRUE, "Writable"=FALSE, "Attribute Name"="CameraInformation::BaseAddress"}, {"Attribute Type"=enum."Enum", "Readable"=TRUE, "Writable"=FALSE, "Attribute Name"="CameraInformation::BusType"}, {"Attribute Type"=enum."String", "Readable"=TRUE, "Writable"=FALSE, "Attribute Name"="CameraInformation::ModelName"}, {"Attribute Type"=enum."String", "Readable"=TRUE, "Writable"=FALSE, "Attribute Name"="CameraInformation::PrimaryURLString"}, {"Attribute Type"=enum."String", "Readable"=TRUE, "Writable"=FALSE, "Attribute Name"="CameraInformation::SecondaryURLString"}, {"Attribute Type"=enum."U32", "Readable"=TRUE, "Writable"=FALSE, "Attribute Name"="CameraInformation::SerialNumberHigh"}, {"Attribute Type"=enum."U32", "Readable"=TRUE, "Writable"=FALSE, "Attribute Name"="CameraInformation::SerialNumberLow"}, {"Attribute Type"=enum."Enum", "Readable"=TRUE, "Writable"=FALSE, "Attribute Name"="CameraInformation::USBConnectionSpeed"}, {"Attribute Type"=enum."String", "Readable"=TRUE, "Writable"=FALSE, "Attribute Name"="CameraInformation::VendorName"}, {"Attribute Type"=enum."Bool", "Readable"=TRUE, "Writable"=FALSE, "Attribute Name"="StatusInformation::AcqInProgress"}, {"Attribute Type"=enum."I64", "Readable"=TRUE, "Writable"=FALSE, "Attribute Name"="StatusInformation::HandledEventCount"}, {"Attribute Type"=enum."I64", "Readable"=TRUE, "Writable"=FALSE, "Attribute Name"="StatusInformation::IncompleteBufferCount"}, {"Attribute Type"=enum."I64", "Readable"=TRUE, "Writable"=FALSE, "Attribute Name"="StatusInformation::LastBufferCount"}, {"Attribute Type"=enum."U32", "Readable"=TRUE, "Writable"=FALSE, "Attribute Name"="StatusInformation::LastBufferNumber"}, {"Attribute Type"=enum."I64", "Readable"=TRUE, "Writable"=FALSE, "Attribute Name"="StatusInformation::LostBufferCount"}, {"Attribute Type"=enum."I64", "Readable"=TRUE, "Writable"=FALSE, "Attribute Name"="StatusInformation::LostEventCount"}]
  out "ValueString":string
  out "Array of writeable attributes":string[](array[string])=["Name:\"AcquisitionAttributes::Bayer::Algorithm\",Type:\"Enum\",Value:\"Bilinear\"", "Name:\"AcquisitionAttributes::Bayer::GainB\",Type:\"DBL\",Value:\"1\"", "Name:\"AcquisitionAttributes::Bayer::GainG\",Type:\"DBL\",Value:\"1\"", "Name:\"AcquisitionAttributes::Bayer::GainR\",Type:\"DBL\",Value:\"1\"", "Name:\"AcquisitionAttributes::Bayer::Pattern\",Type:\"Enum\",Value:\"Use hardware value\"", "Name:\"CameraAttributes::Brightness::Mode\",Type:\"Enum\",Value:\"UnknownEnumValue\"", "Name:\"CameraAttributes::Brightness::Value\",Type:\"I64\",Value:\"0\"", "Name:\"CameraAttributes::Exposure::Mode\",Type:\"Enum\",Value:\"UnknownEnumValue\"", "Name:\"CameraAttributes::Exposure::Value\",Type:\"DBL\",Value:\"0.015625\"", "Name:\"CameraAttributes::Gain::Mode\",Type:\"Enum\",Value:\"UnknownEnumValue\"", "Name:\"CameraAttributes::Gain::Value\",Type:\"I64\",Value:\"0\"", "Name:\"AcquisitionAttributes::Height\",Type:\"U32\",Value:\"1024\"", "Name:\"AcquisitionAttributes::OutputImageType\",Type:\"Enum\",Value:\"Auto\"", "Name:\"AcquisitionAttributes::PayloadSize\",Type:\"U32\",Value:\"2621440\"", "Name:\"AcquisitionAttributes::PixelFormat\",Type:\"Enum\",Value:\"BGRA 8 Packed\"", "Name:\"AcquisitionAttributes::Timeout\",Type:\"U32\",Value:\"5000\"", "Name:\"AcquisitionAttributes::VerticalMirror\",Type:\"Bool\",Value:\"false\"", "Name:\"AcquisitionAttributes::VideoMode\",Type:\"Enum\",Value:\"1280x1024 YUY2 42.39fps\"", "Name:\"AcquisitionAttributes::Width\",Type:\"U32\",Value:\"1280\"", "Name:\"CameraInformation::BusType\",Type:\"Enum\",Value:\"DirectShow\"", "Name:\"CameraInformation::ModelName\",Type:\"String\",Value:\"\"", "Name:\"CameraInformation::SerialNumberHigh\",Type:\"U32\",Value:\"3674102481\"", "Name:\"CameraInformation::SerialNumberLow\",Type:\"U32\",Value:\"4032829644\"", "Name:\"CameraInformation::VendorName\",Type:\"String\",Value:\"Basler GenICam Source\"", "Name:\"StatusInformation::AcqInProgress\",Type:\"Bool\",Value:\"false\"", "Name:\"StatusInformation::LastBufferCount\",Type:\"I64\",Value:\"0\"", "Name:\"StatusInformation::LastBufferNumber\",Type:\"U32\",Value:\"4294967292\"", "Name:\"StatusInformation::LostBufferCount\",Type:\"I64\",Value:\"0\""]
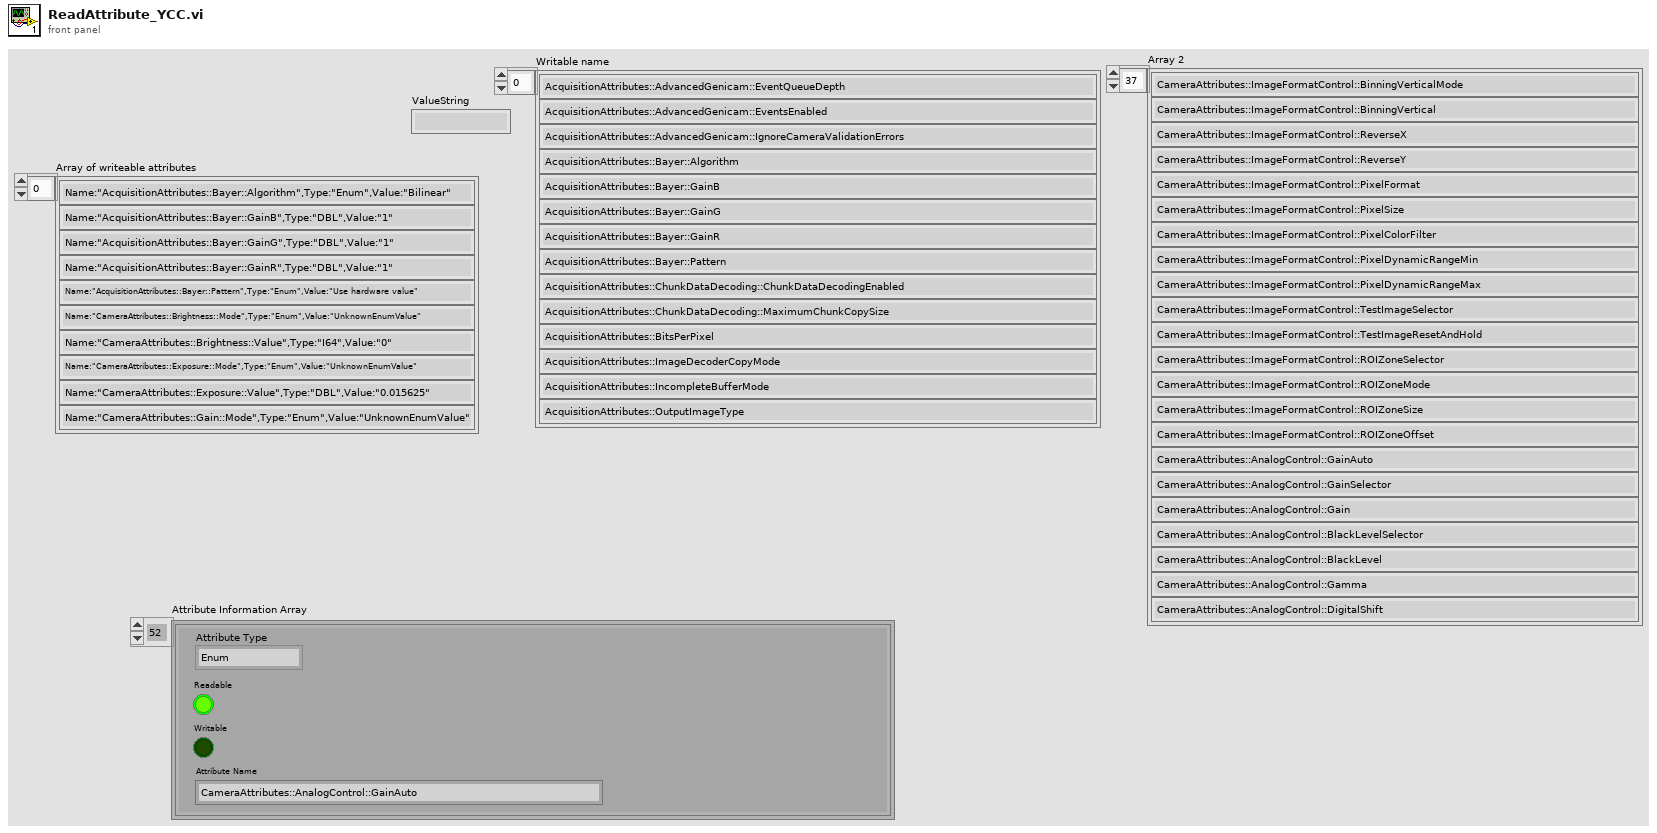
[diagram p1: front panel]
types:
  T1 = typedef "NI_Vision_Acquisition_Software.lvlib/IMAQdx Attribute Type.ctl" = enum32{"U32", "I64", "DBL", "String", "Enum", "Bool", "Command"}
  T2 = cluster{"Attribute Type":T1, "Readable":bool, "Writable":bool, "Attribute Name":string}[]
  T3 = typedef "NI_Vision_Acquisition_Software.lvlib/IMAQdx Camera Control Mode.ctl" = enum32{"Controller", "Listener"}
  T4 = typedef "IMAQdx.ctl" = refnum<k21>
  T5 = typedef "NI_Vision_Acquisition_Software.lvlib/IMAQdx Attribute Visibility.ctl" = enum32{"Simple", "Intermediate", "Advanced"}
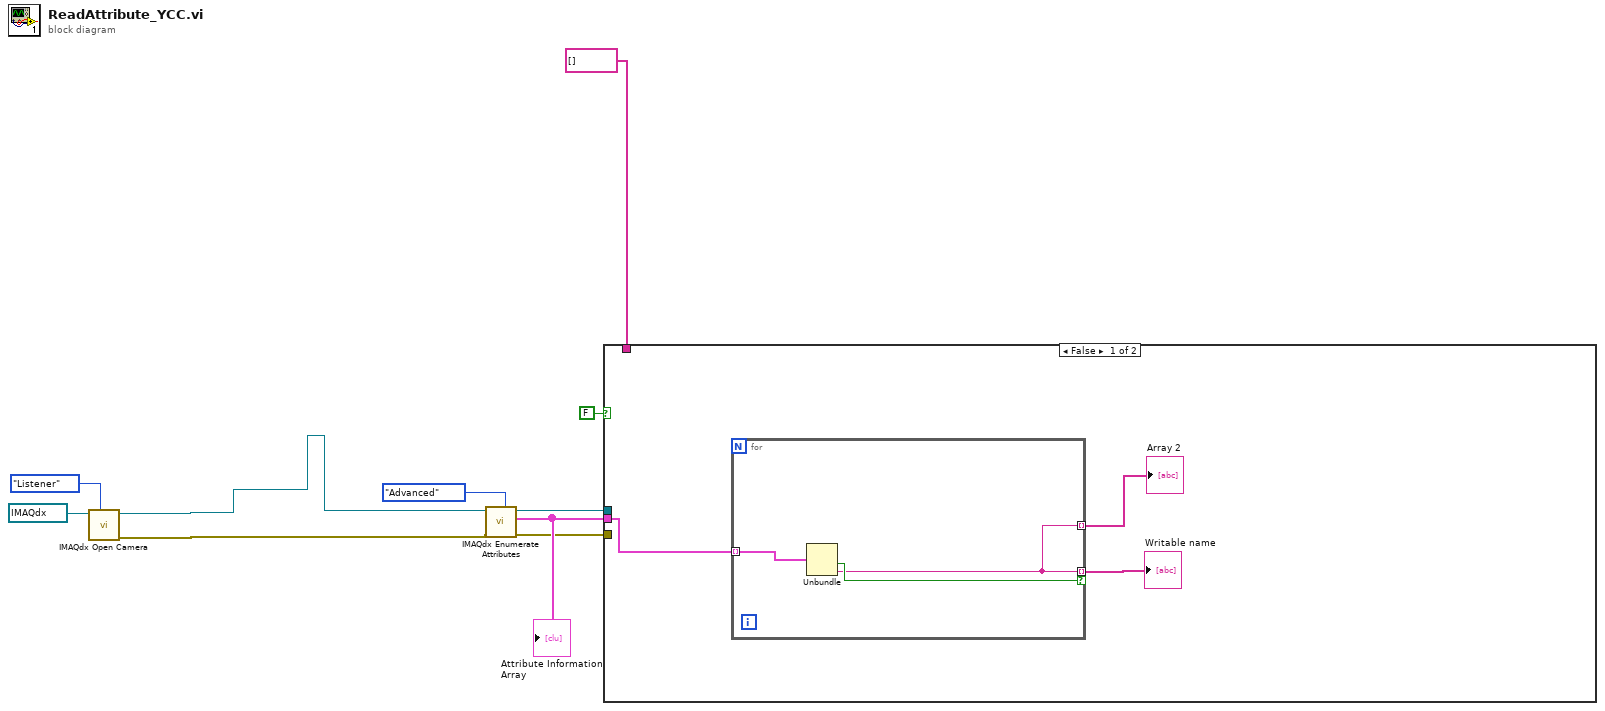
[diagram p0: block diagram]
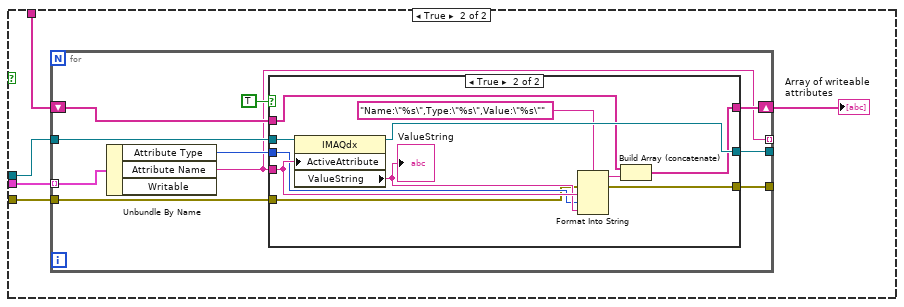
[diagram p2: hidden frame]
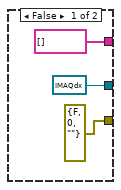
[diagram p3: hidden frame]
diagram:
  n1 = call <vilib>:"IMAQdx Open Camera.vi"("Camera Control Mode"=IMAQdx_Camera_Control_Mode."Listener", "Session In"=T4 "cam2") -> ("error out"=w3:errorcluster, "Session Out"=w4:T4)  [unwired: 8 in]
  n2 = call <vilib>:"IMAQdx Enumerate Attributes.vi"("Visibility"=IMAQdx_Attribute_Visibility."Advanced", "error in"=w3, "Session In"=w4) -> ("error out"=w7:errorcluster, "Attribute Information Array"=w9:T2, "Session Out"=w6:T4)  [unwired: 6 in]
  "Attribute Information Array" <- w9
  n3 = case shown="False" FALSE {
    tunnel: w9 -> [w13 w21]
    tunnel: string[] [] -> [_ w20]
    tunnel: w7 -> [_ w18]
    tunnel: w6 -> [_ w17]
    frame False {
      n4 = for {
        tunnel: w13 -> [w16] mode=indexing
        tunnel: [w14] -> w12 mode=indexing if=w15
        tunnel: [w14] -> w11 mode=indexing
        n5 = Unbundle(w16) -> ("Writable"=w15:bool, "Attribute Name"=w14:string)  [unwired: 2 out]
      }
      "Writable name" <- w12
      "Array 2" <- w11
    }
    frame True {
      n6 = for {
        tunnel: w21 -> [w31] mode=indexing
        shift-right: [w27] -> w19
        shift-left: w20 -> [w26]
        tunnel: w18 -> [w25]
        tunnel: [w24] -> _
        tunnel: [w22] -> _ mode=indexing
        tunnel: w17 -> [w30]
        tunnel: [w29] -> _
        n7 = Unbundle By Name(w31) -> ("Attribute Type"=w28:T1, "Attribute Name"=w22:string)  [unwired: 1 out]
        n8 = case shown="True" TRUE {
          tunnel: w30 -> [_ w45]
          tunnel: [T4 refnum ("Session Out") w44] -> w29
          tunnel: w22 -> [_ w42]
          tunnel: w28 -> [_ w40]
          tunnel: [string[] [] w38] -> w27
          tunnel: w26 -> [_ w37]
          tunnel: w25 -> [_ w36]
          tunnel: [errorcluster {"status"=FALSE, "code"=0, "source"=""} ("error IO") w35] -> w24
          frame False {
          }
          frame True {
            n9 = property class="IMAQdx"(reference=w45, "ActiveAttribute"=w42) -> (reference out=w44:T4, "ValueString"=w41:string)  [unwired: 1 in, 1 out]
            "ValueString" <- w41
            n10 = Format Into String(format string="Name:\"%s\",Type:\"%s\",Value:\"%s\"", error in=w36, w42, w40, w41) -> (resulting string=w39:string, error out=w35:errorcluster)  [unwired: 1 in]
            n11 = Build Array (concatenate)(w37, w39) -> (w38:string[])
          }
        }
      }
      "Array of writeable attributes" <- w19
    }
  }
